vi "Source-Destination Pairs.vi"() -> (3 "Source-Dest Pairs":T1(array[cluster]))   [LabVIEW 2020, in "slsc-switch-benchmarks.lvlib"]
uses:
  slsc-switch-benchmarks.lvlib
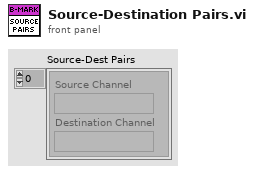
[diagram p1: front panel]
types:
  T1 = cluster{"Source Channel":string, "Destination Channel":string}[]
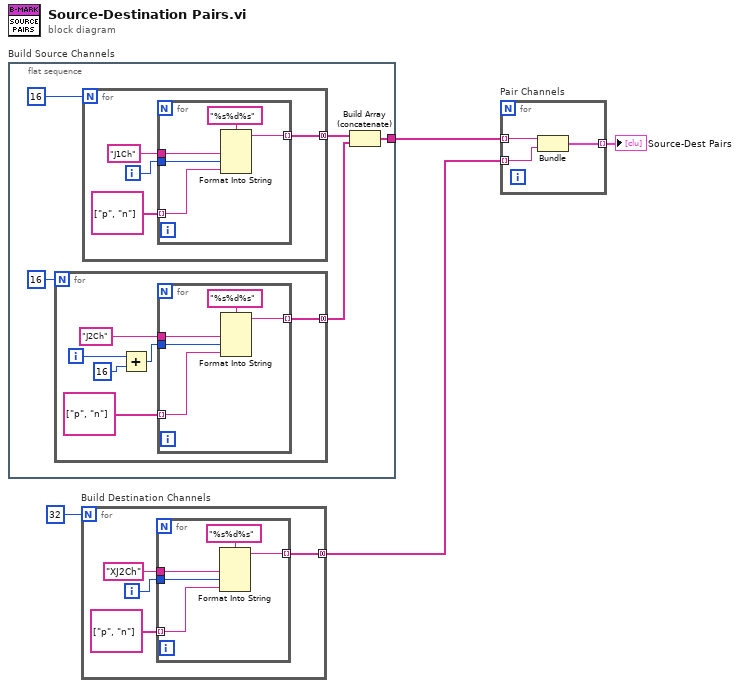
[diagram p0: block diagram]
diagram:
  n1 = flat-sequence "Build Source Channels" {
    tunnel: [w5] -> w3
    frame #0 {
      n2 = for {
        N: 16 -> [_]
        tunnel: [w13] -> w9 mode=concatenating
        i -> [w14]
        n3 = Add(x=w14, y=16) -> (x+y=w11:i32)
        n4 = for {
          tunnel: "J2Ch" -> [w20]
          tunnel: w11 -> [w19]
          tunnel: [w18] -> w13 mode=indexing
          tunnel: string[] ["p", "n"] -> [w17] mode=indexing
          n5 = Format Into String(format string="%s%d%s", w20, w19, w17) -> (resulting string=w18:string)  [unwired: 2 in, 1 out]
        }
      }
      n6 = for {
        N: 16 -> [_]
        tunnel: [w22] -> w8 mode=concatenating
        i -> [w23]
        n7 = for {
          tunnel: "J1Ch" -> [w29]
          tunnel: w23 -> [w28]
          tunnel: [w27] -> w22 mode=indexing
          tunnel: string[] ["p", "n"] -> [w26] mode=indexing
          n8 = Format Into String(format string="%s%d%s", w29, w28, w26) -> (resulting string=w27:string)  [unwired: 2 in, 1 out]
        }
      }
      n9 = Build Array (concatenate)(w8, w9) -> (w5:string[])
    }
  }
  n10 = for "Build Destination Channels" {
    N: 32 -> [_]
    tunnel: [w31] -> w2 mode=concatenating
    i -> [w32]
    n11 = for {
      tunnel: "XJ2Ch" -> [w38]
      tunnel: w32 -> [w37]
      tunnel: [w36] -> w31 mode=indexing
      tunnel: string[] ["p", "n"] -> [w35] mode=indexing
      n12 = Format Into String(format string="%s%d%s", w38, w37, w35) -> (resulting string=w36:string)  [unwired: 2 in, 1 out]
    }
  }
  n13 = for "Pair Channels" {
    tunnel: w3 -> [w41] mode=indexing
    tunnel: w2 -> [w40] mode=indexing
    tunnel: [w39] -> w1 mode=indexing
    n14 = Bundle(w41, w40) -> (w39:cluster{string, string})  [unwired: 1 in]
  }
  "Source-Dest Pairs" <- w1
